vi "Get Cell Value with Range.vi"(4 "error in (no error)":errorcluster caption="错误输入（无错误）", 5 "Excel._Worksheet":refnum<k7>, 6 "Col":i32 caption="列", 7 "Row":i32 caption="行") -> (0 "error out":errorcluster caption="错误输出", 1 "Data Out":variant, 2 "Range":refnum<k7> caption="范围", 3 "Excel._Worksheet":refnum<k7>)   [LabVIEW 2020]
doc: "本VI会将工作表中由“行：列”指定的单元格的值设置为输入“值”。首先将行和列的数值输入转换为Excel格式的A1和B1等，然后执行工作表对象的“范围方法”并设置范围的“值”属性。在循环的每次迭代中都将释放范围的自动化引用句柄。"
panel:
  in  "dummy Range":refnum<k7> caption="虚设范围"
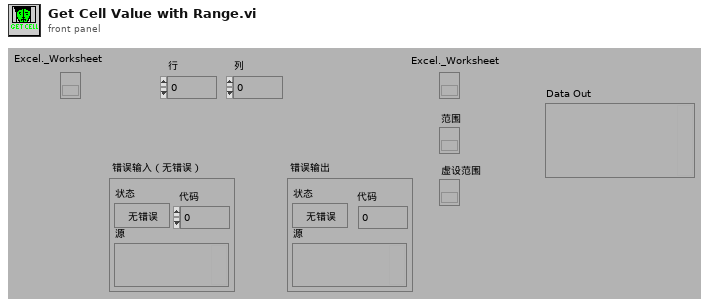
[diagram p1: front panel]
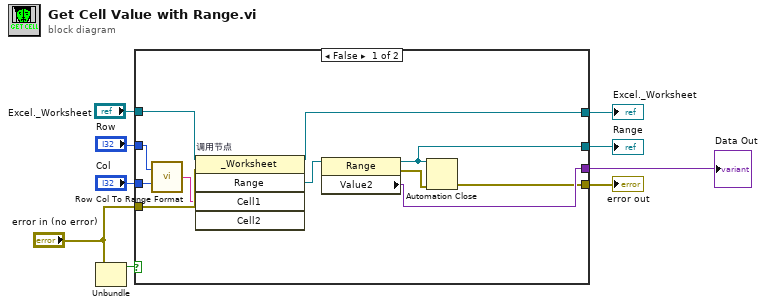
[diagram p0: block diagram]
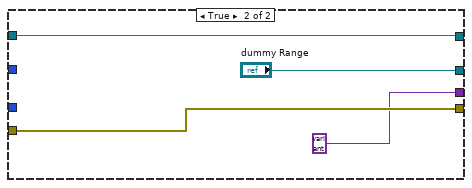
[diagram p2: hidden frame]
diagram:
  n1 = Unbundle("error in (no error)") -> ("status"=w5:bool)  [unwired: 2 out]
  n2 = case shown="False" w5 {
    tunnel: "Col" -> [w20 _]
    tunnel: "Row" -> [w19 _]
    tunnel: "error in (no error)" -> [w14 w24]
    tunnel: [w10 w24] -> w7
    tunnel: [w13 w23] -> w4
    tunnel: "Excel._Worksheet" -> [w16 w23]
    tunnel: [w15 "dummy Range"] -> w2
    tunnel: [w11 variant ("Value2")] -> w1
    frame False {
      n3 = call "Row Col To Range Format.vi"("Column"=w20, "Row"=w19) -> ("Output String"=w12:string)
      n4 = invoke on="调用节点" class="_Worksheet" method="Range"(reference=w16, error in=w14, "Cell1"=w12) -> (reference out=w13:refnum<k7>, "Range"=w18:refnum<k7>)  [unwired: 2 in, 3 out]
      n5 = property class="Range"(reference=w18) -> (reference out=w15:refnum<k7>, error out=w17:errorcluster, "Value2"=w11:variant)  [unwired: 1 in]
      n6 = Automation Close ("关闭自动化")(3:w17, 5:w15) -> (0:w10:errorcluster)
    }
    frame True {
    }
  }
  "Excel._Worksheet" <- w4
  "error out" <- w7
  "Range" <- w2
  "Data Out" <- w1
